vi "Create Fixed Wheel.vi"(6 "motor communication":refnum<class "NI_Robotics_Motor Communication.lvclass">, 8 "error in (no error)":errorcluster, 10 "wheel name":string, 11 "wheel parameters":T1={"wheel radius"=1.0, "gear ratio"=1.0, "forward rotation direction"=0} {"forward rotation direction" items=["Clockwise", "Counterclockwise"]}) -> (0 "error out":errorcluster, 3 "fixed wheel out":refnum<class "NI_Robotics_Fixed Wheel.lvclass">)   [LabVIEW 2017, in "NI_Robotics_Fixed Wheel.lvclass"]
doc: "Creates a wheel of the type you specify that you can add to a steering frame. You must manually select the polymorphic instance to use."
uses:
  <vilib>/robotics/Steering/Fixed Wheel/NI_Robotics_Fixed Wheel.lvclass
  c:/Program Files (x86)/National Instruments/LabVIEW 2017/vi.lib/robotics/Steering/Wheel/NI_Robotics_Wheel.lvclass
  <vilib>/robotics/Steering/Wheel/Wheel Parameters.ctl
  <vilib>/robotics/Steering/Wheel/Rotation Direction.ctl
  <vilib>/robotics/Actuation/Motor Communication/NI_Robotics_Motor Communication.lvclass
  <vilib>/robotics/Actuation/Motor Communication/NI_Robotics_Motor Communication.lvclass/NI_Robotics_Motor Communication.ctl
  <vilib>/robotics/Steering/Wheel/NI_Robotics_Wheel.lvclass/NI_Robotics_Wheel.ctl
  <vilib>/robotics/Actuation/Motor Communication/Get Initialized State.vi
  <vilib>/robotics/Actuation/Motor Communication Val/NI_Robotics_Motor Communication Val.lvclass
  c:/Program Files (x86)/National Instruments/LabVIEW 2017/vi.lib/robotics/Actuation/Motor Communication/NI_Robotics_Motor Communication.lvclass
  <vilib>/robotics/Actuation/Motor Communication Val/Initialize Motor Communication Val.vi
  <vilib>/robotics/Steering/Wheel/NI_Robotics_Wheel.lvclass
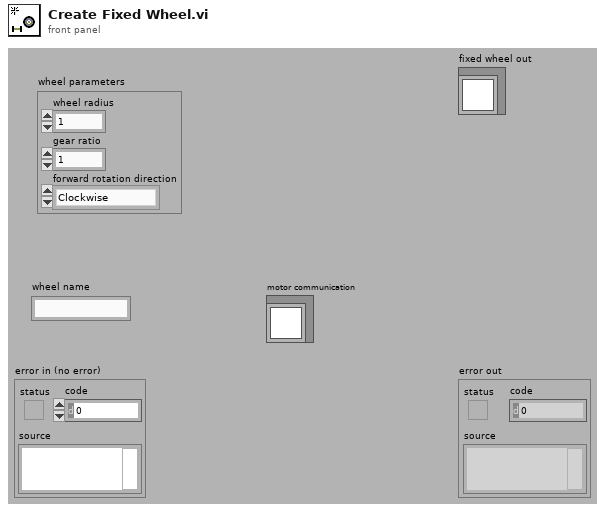
[diagram p1: front panel]
types:
  T1 = typedef "NI_Robotics_Wheel.lvclass/Wheel Parameters.ctl" = cluster{"wheel radius":dbl, "gear ratio":dbl, "forward rotation direction":T2}
  T2 = typedef "NI_Robotics_Wheel.lvclass/Rotation Direction.ctl" = u16
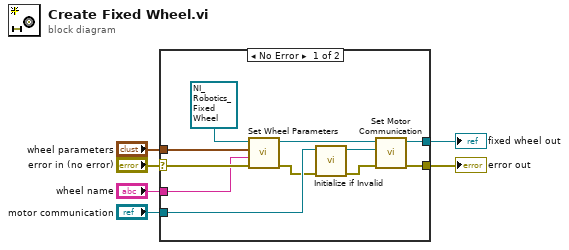
[diagram p0: block diagram]
diagram:
  n1 = case shown="No Error" "error in (no error)" {
    selector: "error in (no error)" -> [w16 w18]
    tunnel: [w11 w18] -> w5
    tunnel: [w12 _] -> w4
    tunnel: "motor communication" -> [w10 _]
    tunnel: "wheel parameters" -> [w15 _]
    tunnel: "wheel name" -> [w14 _]
    frame No Error {
      n2 = call <vilib>:"Set Wheel Parameters.vi"("error in (no error)"=w16, "wheel name"=w14, "wheel parameters"=w15, "wheel in"=refnum<class "NI_Robotics_Fixed Wheel.lvclass"> refnum ("Fixed Wheel in")) -> ("error out"=w8:errorcluster, "wheel out"=w13:refnum<class "NI_Robotics_Fixed Wheel.lvclass">)  [unwired: 6 in]
      n3 = call <vilib>:"Initialize if Invalid.vi"("error in (no error)"=w8, "motor communication in"=w10) -> ("error out"=w7:errorcluster, "motor communication out"=w9:refnum<class "NI_Robotics_Motor Communication.lvclass">)  [unwired: 7 in, 1 out]
      n4 = call <vilib>:"Set Motor Communication.vi"("error in (no error)"=w7, "motor communication"=w9, "wheel in"=w13) -> ("error out"=w11:errorcluster, "wheel out"=w12:refnum<class "NI_Robotics_Fixed Wheel.lvclass">)  [unwired: 7 in]
    }
    frame Error {
    }
  }
  "error out" <- w5
  "fixed wheel out" <- w4
